vi "Set Text.vi"(8 "error in (no error)":errorcluster caption="entrée d'erreur (pas d'erreur)", 10 "Text":string, 11 "Class File (Default) en entrée":refnum<class "Class File (Default).lvclass">) -> (0 "error out":errorcluster caption="sortie d'erreur", 3 "Class File (Default) en sortie":refnum<class "Class File (Default).lvclass">)   [LabVIEW 2020, in "Library Instrument & Equipement.lvlib" / "Library File.lvlib" / "Class File (Default).lvclass"]
uses:
  Class File (Default).lvclass
  Class File (Default).lvclass/Class File (Default).ctl
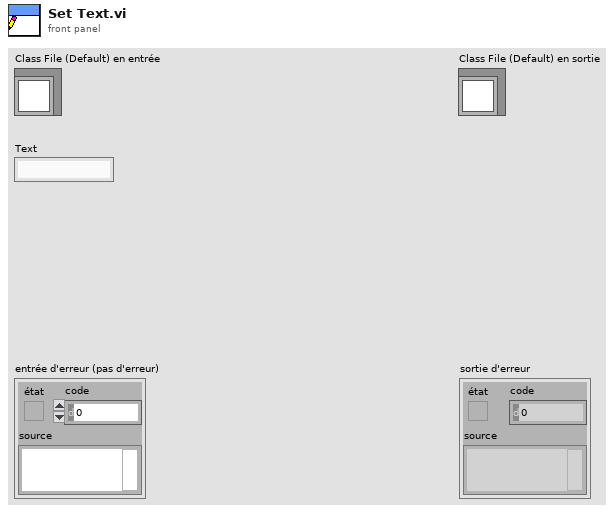
[diagram p1: front panel]
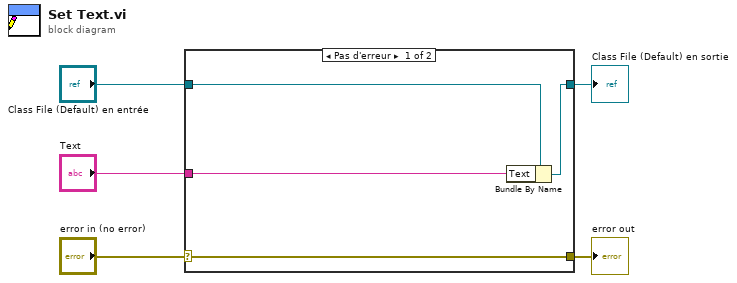
[diagram p0: block diagram]
diagram:
  n1 = case shown="Pas d'erreur" "error in (no error)" {
    selector: "error in (no error)" -> [w9 w10]
    tunnel: [w9 w10] -> w4
    tunnel: [w7 w11] -> w2
    tunnel: "Class File (Default) en entrée" -> [w8 w11]
    tunnel: "Text" -> [w6 _]
    frame No Error {
      n2 = Bundle By Name(cluster=w8, "Text"=w6) -> (w7:refnum<class "Class File (Default).lvclass">)
    }
    frame Error {
    }
  }
  "error out" <- w4
  "Class File (Default) en sortie" <- w2
